vi "Main.vi"() -> ()   [LabVIEW 2017]
uses:
  shared/Kobuki Sensor Display.ctl
  controls/StatesEnum.ctl
  <vilib>/Platform/TimedLoop/XDataNode/timing_clust.ctl
  <vilib>/Platform/TimedLoop/XDataNode/nitl_modes.ctl
  <vilib>/Platform/TimedLoop/XDataNode/wakeup.ctl
  shared/Sensors.ctl
  shared/Accelerometer.ctl
  Kobuki/KobukiSensors.ctl
  Kobuki/Kobuki Bumps and WheelDrops.ctl
  Kobuki/Kobuki Buttons.ctl
  <vilib>/myRIO/Common/Instrument Driver Framework/myRIO v1.0/UART/vis/myRIO v1.0 Close UART.vi
  <vilib>/myRIO/Common/Instrument Driver Framework/myRIO v1.0/myRIO v1.1 Open.vi
  <vilib>/myRIO/Common/Instrument Driver Framework/Utilities/vis/FPGA Ref Manager.vi
  <vilib>/myRIO/Common/Instrument Driver Framework/myRIO v1.0/myRIO v1.0 Reset FPGA.vi
  <vilib>/myRIO/Common/Instrument Driver Framework/myRIO v1.0/IRQ/vis/myRIO v1.0 IRQ Info FGV.vi
  <vilib>/myRIO/Common/Instrument Driver Framework/myRIO v1.0/IRQ/vis/myRIO v1.0 Timer IRQ Info FGV.vi
  <vilib>/myRIO/Common/Instrument Driver Framework/myRIO v1.0/IRQ/vis/myRIO v1.0 ISR Agent.vi
  <vilib>/platform/TimedLoop/XDataNode/XDataNode.xnode
  <vilib>/myRIO/Instrument Drivers/Utilities/Utilities.lvlib
  <vilib>/Platform/TimedLoop/XDataNode/XDNodeRunTimeDep.lvlib
panel:
  in  "Tab Control":T1(tab)
  out "Kobuki Sensors (graphical)":T2 {"Right Wheel (mm/s)" scale=-500.0..500.0; "Left Wheel (mm/s)" scale=-500.0..500.0}
  out "Charge Status":i8(ring) items=["DISCHARGING"=0, "DOCKING_CHARGED"=2, "DOCKING_CHARGING"=6, "ADAPTER_CHARGED"=18, "ADAPTER_CHARGING"=22]
  out "Kobuki Battery Voltage":dbl(knob)=12000.0 scale=12.0..16.4 scale format="%#.1f"
  out "CurrentState":T4=enum."Init"
  out "Loop Duration":i64
  out "error out":errorcluster
  in  "stop":bool
  out "Target Running":bool
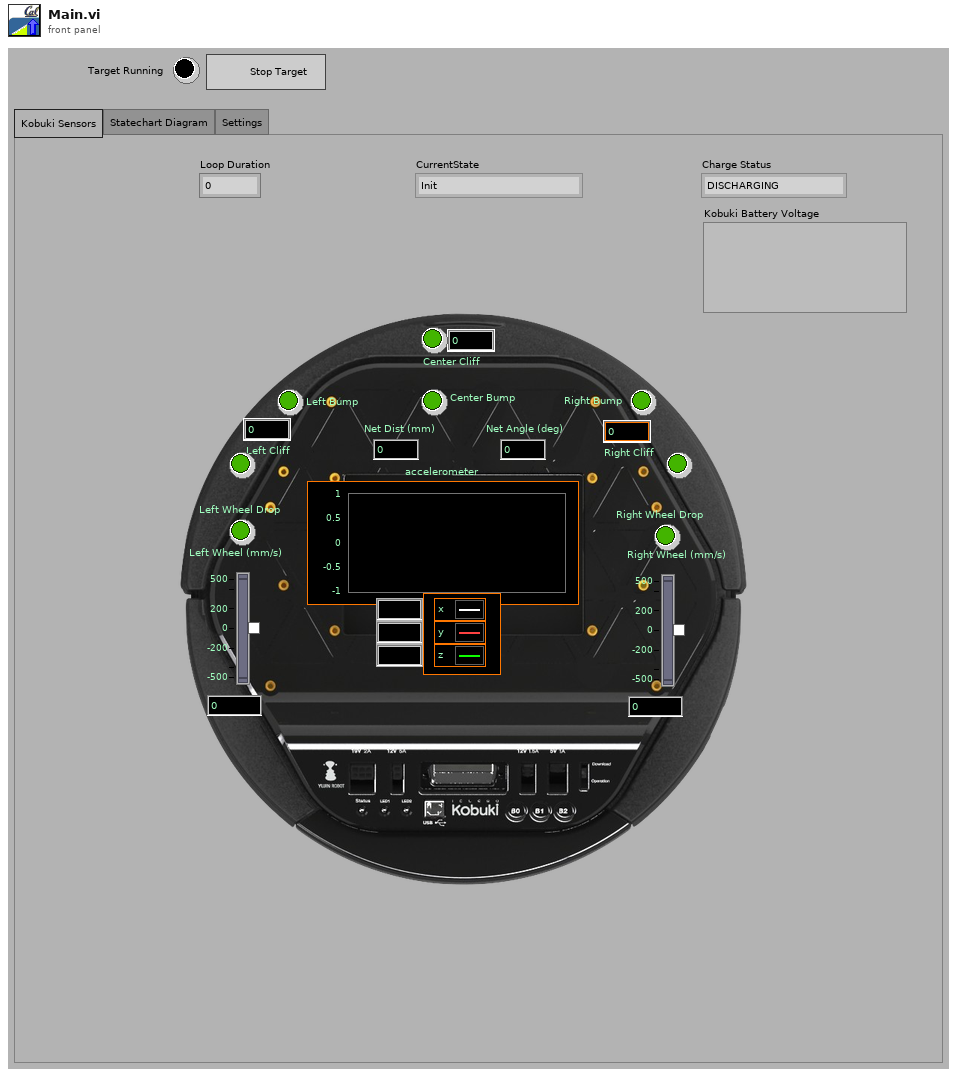
[diagram p1: front panel]
types:
  T1 = enum32{"Kobuki Sensors", "Statechart Diagram", "Settings"}
  T2 = typedef "Kobuki Sensor Display.ctl" = cluster{"Center Bump":bool, "Left Wheel Drop":bool, "Right Wheel Drop":bool, "Left Bump":bool, "Right Bump":bool, "Left Cliff":bool, "Center Cliff":bool, "Right Cliff":bool, "Net Dist (mm)":i32, "Net Angle (deg)":i32, "Left Cliff":u16, "Center Cliff":u16, "Right Cliff":u16, "  Left Wheel (mm/s)":i16, "Right Wheel (mm/s)":i16, "accelerometer":T3}
  T3 = typedef "Accelerometer.ctl" = cluster{"x axis (g)":dbl, "y axis (g)":dbl, "z axis (g)":dbl}
  T4 = typedef "StatesEnum.ctl" = enum16{"Run", "Pause", "Init", "Shut"}
  T5 = typedef "XDNodeRunTimeDep.lvlib/timing_clust.ctl" = cluster{"Expected End [f-1]":u64, "Actual End [f-1]":u64, "Finished Late? [f-1]":bool, "Expected End [i-1]":u64, "Actual End [i-1]":u64, "Finished Late? [i-1]":bool, "Expected Start [i]":u64, "Actual Start [i]":u64, "Expected Start [f]":u64, "Actual Start [f]":u64, "Source Name":string, "Structure Name":string, "Period":i64, "Deadline":i64, "Offset":i64, "Start":i64, "Priority":i32, "Timeout":i32, "Mode":T6, "Wakeup Reason":T7, "Error":errorcluster, "Source Type":string, "Secondary Source Type":string, "Global End Time":u64, "Global Start Time":u64, "Frame Duration":u64, "Iteration Duration":u64, "Assigned CPU":i32, "I/O Scan Engine Mode":u32}
  T6 = typedef "XDNodeRunTimeDep.lvlib/nitl_modes.ctl" = enum32{"No Change", "Process missed periods, maintain original phase", "Discard missed periods, maintain original phase", "Process missed periods, ignore original phase", "Discard missed periods, ignore original phase"}
  T7 = typedef "XDNodeRunTimeDep.lvlib/wakeup.ctl" = enum32{"Normal", "Aborted", "Asynchronous wakeup", "Timing source error", "Timed loop error", "Timeout"}
  T8 = typedef "Sensors.ctl" = cluster{"net distance (mm)":i32, "net angle (deg)":i32, "accelerometer":T3, "Is Simulator?":bool, "Kobuki Sensors":T9, "Requested Left Wheel Velocity(mm/s)":i32, "Requested Right Wheel Velocity(mm/s)":i32}
  T9 = typedef "KobukiSensors.ctl" = cluster{"Bumps + Wheel Drops":T10, "Cliff Left":bool, "Cliff Center":bool, "Cliff Right":bool, "Cliff Left Signal":u16, "Cliff Center Signal":u16, "Cliff Right Signal":u16, "Buttons":T11, "Left Wheel Encoder (ticks)":u16, "Right Wheel Encoder (ticks) ":u16, "Left  Wheel PWM":i8, "Right Wheel PWM":i8, "Left Wheel OverCurrent":bool, "Right Wheel OverCurrent ":bool, "Right Wheel Current (x10mA)":i16, "Left  Wheel Current  (x10mA)":i16, "TimeStamp":u16, "Battery Voltage":dbl, "Angle( of 100deg)":i16, "Angle Rate( of 100 deg/sec)":i16, "Charger Source ":i8}
  T10 = typedef "Kobuki Bumps and WheelDrops.ctl" = cluster{"Wheeldrop Left":bool, "Wheeldrop Right":bool, "Bump Left":bool, "Bump Center":bool, "Bump Right":bool}
  T11 = typedef "Kobuki Buttons.ctl" = cluster{"B0":bool, "B1":bool, "B2":bool}
  T12 = typedef "Outputs.ctl" = cluster{"Left Wheel Speed (mm/s)":i16, "Right Wheel Speed (mm/s)":i16}
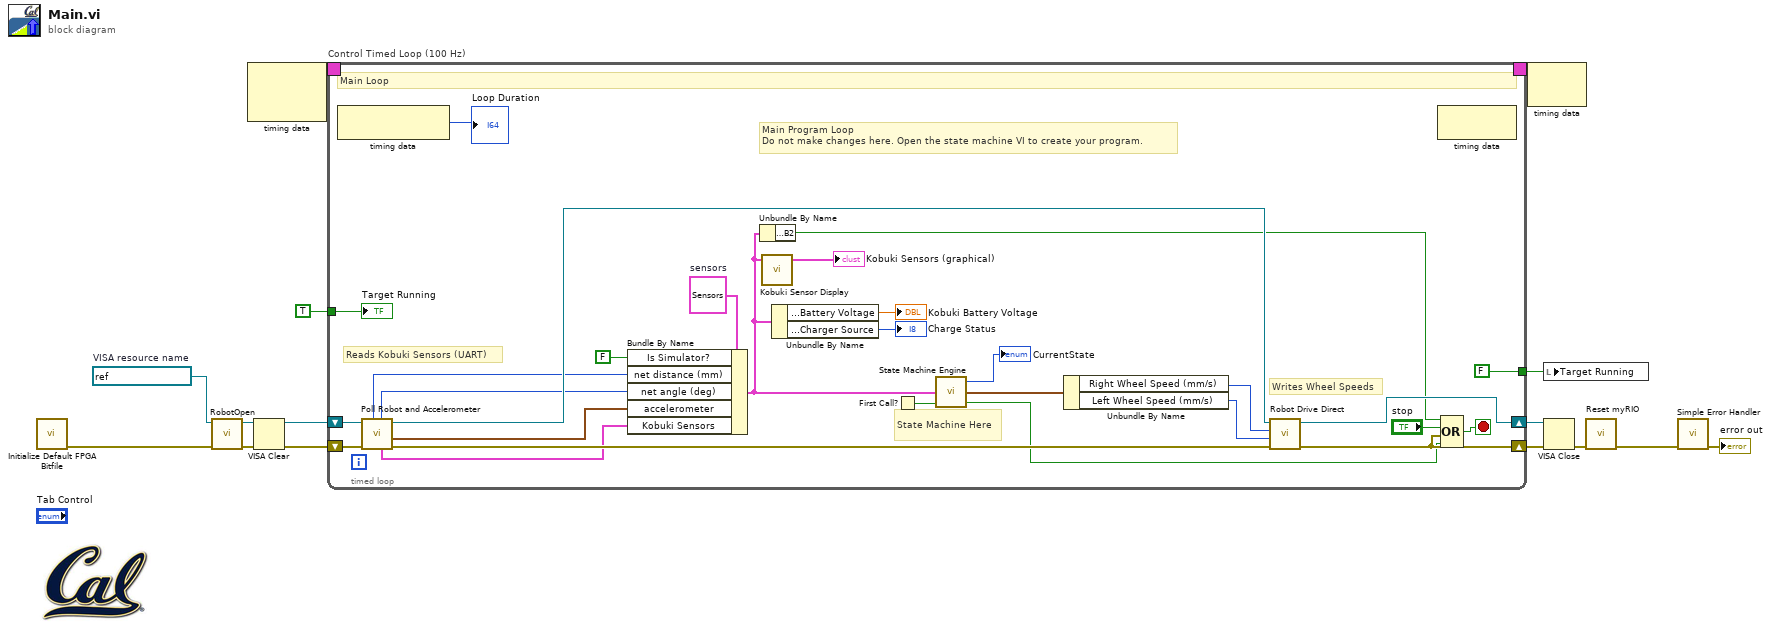
[diagram p0: block diagram]
diagram:
  w12 = refnum<visa-resource-name> "ASRL3::INSTR"  # VISA resource name
  n1 = call <vilib>:"Initialize Default FPGA Bitfile.vi"() -> ("error out"=w10:errorcluster)  [unwired: 11 in]
  n2 = call "RobotOpen.vi"("error in (no error)"=w10, "Robot Communication port name"=w12) -> ("error out"=w8:errorcluster, "Robot Communication port name out"=w15:refnum<visa-resource-name>)  [unwired: 8 in]
  n3 = node-c288() -> (w2:T5)  [unwired: 2 in]
  n4 = VISA Clear(VISA resource name=w15, error in (no error)=w8) -> (VISA resource name out=w6:refnum<visa-resource-name>, error out=w7:errorcluster)
  n5 = timed-loop "Control Timed Loop (100 Hz)" {
    shift-right: [w43] -> w4
    shift-left: w6 -> [w40]
    shift-right: [w26] -> w5
    shift-left: w7 -> [w39]
    tunnel: TRUE ("stop") -> [w34]
    tunnel: [FALSE ("stop")] -> w13
    timing: w2 -> [_]
    timing-out: [_] -> w1
    stop <- w42 stop-if-true
    w29 = T8 {"net distance (mm)"=0, "net angle (deg)"=0, "accelerometer"={"x axis (g)"=0.0, "y axis (g)"=0.0, "z axis (g)"=0.0}, "Is Simulator?"=FALSE, "Kobuki Sensors"={"Bumps + Wheel Drops"={"Wheeldrop Left"=FALSE, "Wheeldrop Right"=FALSE, "Bump Left"=FALSE, "Bump Center"=FALSE, "Bump Right"=FALSE}, "Cliff Left"=FALSE, "Cliff Center"=FALSE, "Cliff Right"=FALSE, "Cliff Left Signal"=0, "Cliff Center Signal"=0, "Cliff Right Signal"=0, "Buttons"={"B0"=FALSE, "B1"=FALSE, "B2"=FALSE}, "Left Wheel Encoder (ticks)"=0, "Right Wheel Encoder (ticks) "=0, "Left  Wheel PWM"=0, "Right Wheel PWM"=0, "Left Wheel OverCurrent"=FALSE, "Right Wheel OverCurrent "=FALSE, "Right Wheel Current (x10mA)"=0, "Left  Wheel Current  (x10mA)"=0, "TimeStamp"=0, "Battery Voltage"=0.0, "Angle( of 100deg)"=0, "Angle Rate( of 100 deg/sec)"=0, "Charger Source "=0}, "Requested Left Wheel Velocity(mm/s)"=0, "Requested Right Wheel Velocity(mm/s)"=0}  # sensors
    # "Main Program Loop\nDo not make changes here. Open the state machine VI to create your program."
    # "Writes Wheel Speeds"
    # "Reads Kobuki Sensors (UART)"
    # "State Machine Here"
    # "Main Loop"
    n6 = node-c288() -> (→"Loop Duration":i64)  [unwired: 1 in]
    n7 = call "Poll Robot and Accelerometer.vi"("error in"=w39, "UART in"=w40) -> ("error out"=w38:errorcluster, "Acceleration (g)"=w31:T3, "UART out"=w37:refnum<visa-resource-name>, "Kobuki Sensors  out"=w28:T9, "net angle (deg)"=w35:i32, "net distance (mm)"=w36:i32)  [unwired: 4 in]
    n8 = Bundle By Name(cluster=w29, "Is Simulator?"=FALSE, "net distance (mm)"=w36, "net angle (deg)"=w35, "accelerometer"=w31, "Kobuki Sensors"=w28) -> (w16:T8)
    n9 = Unbundle By Name(w16) -> ("Kobuki Sensors.Buttons.B2"=w32:bool)
    n10 = call "Kobuki Sensor Display.vi"("sensors"=w16) -> ("Kobuki Sensors Display"=→"Kobuki Sensors (graphical)":T2)  [unwired: 4 in]
    n11 = Unbundle By Name(w16) -> ("Kobuki Sensors.Battery Voltage"=→"Kobuki Battery Voltage":dbl, "Kobuki Sensors.Charger Source"=→"Charge Status":i8)
    n12 = First Call?() -> (First Call?: T/F=w18:bool)
    n13 = call "State Machine Engine.vi"("Init?"=w18, "Inputs"=w16) -> ("Terminated?"=w17:bool, "Outputs"=w22:T12, "CurrentState"=→"CurrentState":T4)  [unwired: 1 in]
    n14 = Unbundle By Name(w22) -> ("Right Wheel Speed (mm/s)"=w24:i16, "Left Wheel Speed (mm/s)"=w23:i16)
    n15 = call "Robot Drive Direct.vi"("error in"=w38, "Left Wheel Velocity (mm/s)"=w23, "Right Wheel Velocity (mm/s)"=w24, "UART port in"=w37) -> ("error out"=w26:errorcluster, "UART port out"=w43:refnum<visa-resource-name>)  [unwired: 6 in]
    n16 = node-c288() -> ()  [unwired: 1 in, 1 out]
    n17 = Compound Arithmetic op=OR(w32, "stop", w26, w17) -> (w42:bool)
    "Target Running" <- w34
  }
  n18 = node-c288(w1) -> ()  [unwired: 1 out]
  n19 = local write "Target Running"(w13) -> ()
  n20 = VISA Close(VISA resource name=w4, error in (no error)=w5) -> (error out=w3:errorcluster)
  n21 = call <vilib>:"Reset myRIO.vi"("error in (no error)"=w3) -> ("error out"=w11:errorcluster)  [unwired: 10 in]
  n22 = call <vilib>:"Simple Error Handler.vi"("error in (no error)"=w11) -> ("error out"=→"error out":errorcluster)  [unwired: 4 in, 4 out]
